vi "EVS Main.vi"() -> ()   [LabVIEW 2009]
uses:
  TypeDefs/cRIO-EVS Comm/EVS to cRIO UDP packet.ctl
  UDP Lib/UDP Network Location.ctl
  <vilib>/vision/driver/NI_Vision_Acquisition_Software.lvlib
  <vilib>/NI_Real-Time Target Support.lvlib
  <vilib>/Platform/TimedLoop/XDataNode/XDataNode.xnode
  <vilib>/Platform/TimedLoop/XDataNode/timing_clust.ctl
  <vilib>/Platform/TimedLoop/XDataNode/XDNodeRunTimeDep.lvlib
  <vilib>/Platform/TimedLoop/XDataNode/wakeup.ctl
  <vilib>/Platform/TimedLoop/XDataNode/nitl_modes.ctl
  <vilib>/vision/driver/IMAQdx.llb/IMAQdx Acquisition Mode.ctl
  <vilib>/Platform/TimedLoop/XDataNode/loadlvalarms.vi
  <vilib>/userDefined/High Color/IMAQdx.ctl
panel:
  out "Original":T1(plugin-control)
  out "Extracted":T1(plugin-control)
  out "Ramp?":bool
  out "Iteration Duration":i64
  out "Number of ramp regions (left)":i32
  out "Number of ramp regions (right)":i32
  out "Sick array":u16[](array[numeric])
  in  "stop":bool
  out "HB":bool
  in  "IMAQdx Session Left":T2="lcam" caption="Left Session"
  in  "IMAQdx Session Right":T2="rcam" caption="Right Session"
  # "0: Original\n1: Extracted\n2: Masked"
  # "0: Old line extraction\n1: Solid white line (ramp)\n2: LPF"
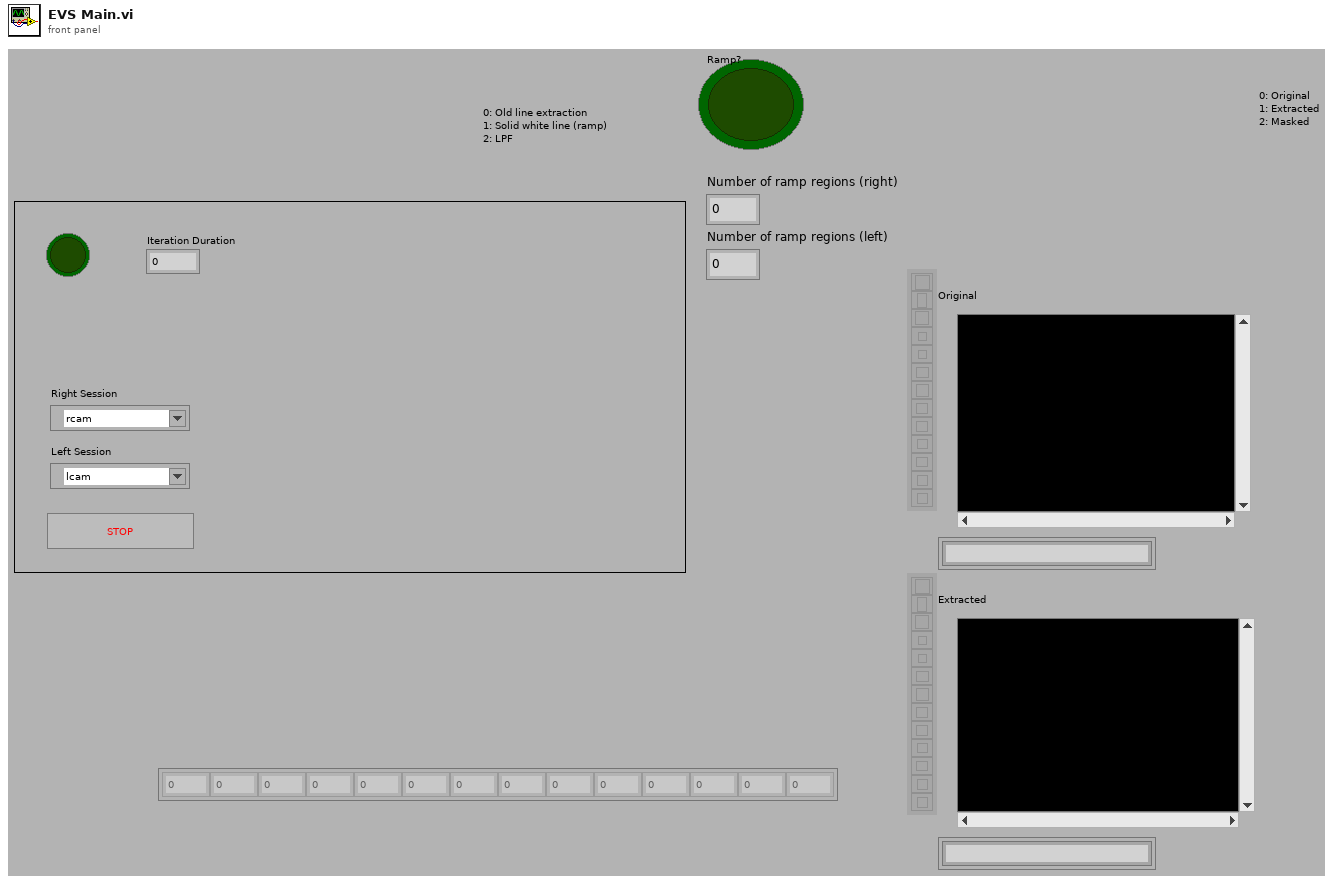
[diagram p1: front panel]
types:
  T1 = typedef "IMAQ Image.ctl" = refnum<image>
  T2 = typedef "IMAQdx.ctl" = refnum<k21>
  T3 = typedef "EVS to cRIO UDP packet.ctl" = cluster{"Camera SICK":u16[], "Camera init":bool, "Array":cluster{"X Coord":void[], "Y Coord":void[]}[]}
  T4 = typedef "NI_Vision_Acquisition_Software.lvlib/IMAQdx Acquisition Mode.ctl" = enum32{"One Shot", "Continuous"}
  T5 = typedef "XDNodeRunTimeDep.lvlib/timing_clust.ctl" = cluster{"Expected End [f-1]":u64, "Actual End [f-1]":u64, "Finished Late? [f-1]":bool, "Expected End [i-1]":u64, "Actual End [i-1]":u64, "Finished Late? [i-1]":bool, "Expected Start [i]":u64, "Actual Start [i]":u64, "Expected Start [f]":u64, "Actual Start [f]":u64, "Source Name":string, "Structure Name":string, "Period":i64, "Deadline":i64, "Offset":i64, "Start":i64, "Priority":i32, "Timeout":i32, "Mode":T6, "Wakeup Reason":T7, "Error":errorcluster, "Source Type":string, "Secondary Source Type":string, "Global End Time":u64, "Global Start Time":u64, "Frame Duration":u64, "Iteration Duration":u64, "Assigned CPU":i32, "I/O Scan Engine Mode":u32}
  T6 = typedef "XDNodeRunTimeDep.lvlib/nitl_modes.ctl" = enum32{"No Change", "Process missed periods, maintain original phase", "Discard missed periods, maintain original phase", "Process missed periods, ignore original phase", "Discard missed periods, ignore original phase"}
  T7 = typedef "XDNodeRunTimeDep.lvlib/wakeup.ctl" = enum32{"Normal", "Aborted", "Asynchronous wakeup", "Timing source error", "Timed loop error", "Timeout"}
  T8 = typedef "UDP Network Location.ctl" = cluster{"IP Address":string, "Port":u16}
  T9 = typedef "UDP Base.ctl" = cluster{"UDP Session":refnum<k16>, "UDP Socket Params":T10}
  T10 = typedef "UDP Socket Params.ctl" = cluster{"Local Port":u16, "Read Timeout":i32, "Write Timeout":i32}
  T11 = typedef "Image Type" = u32
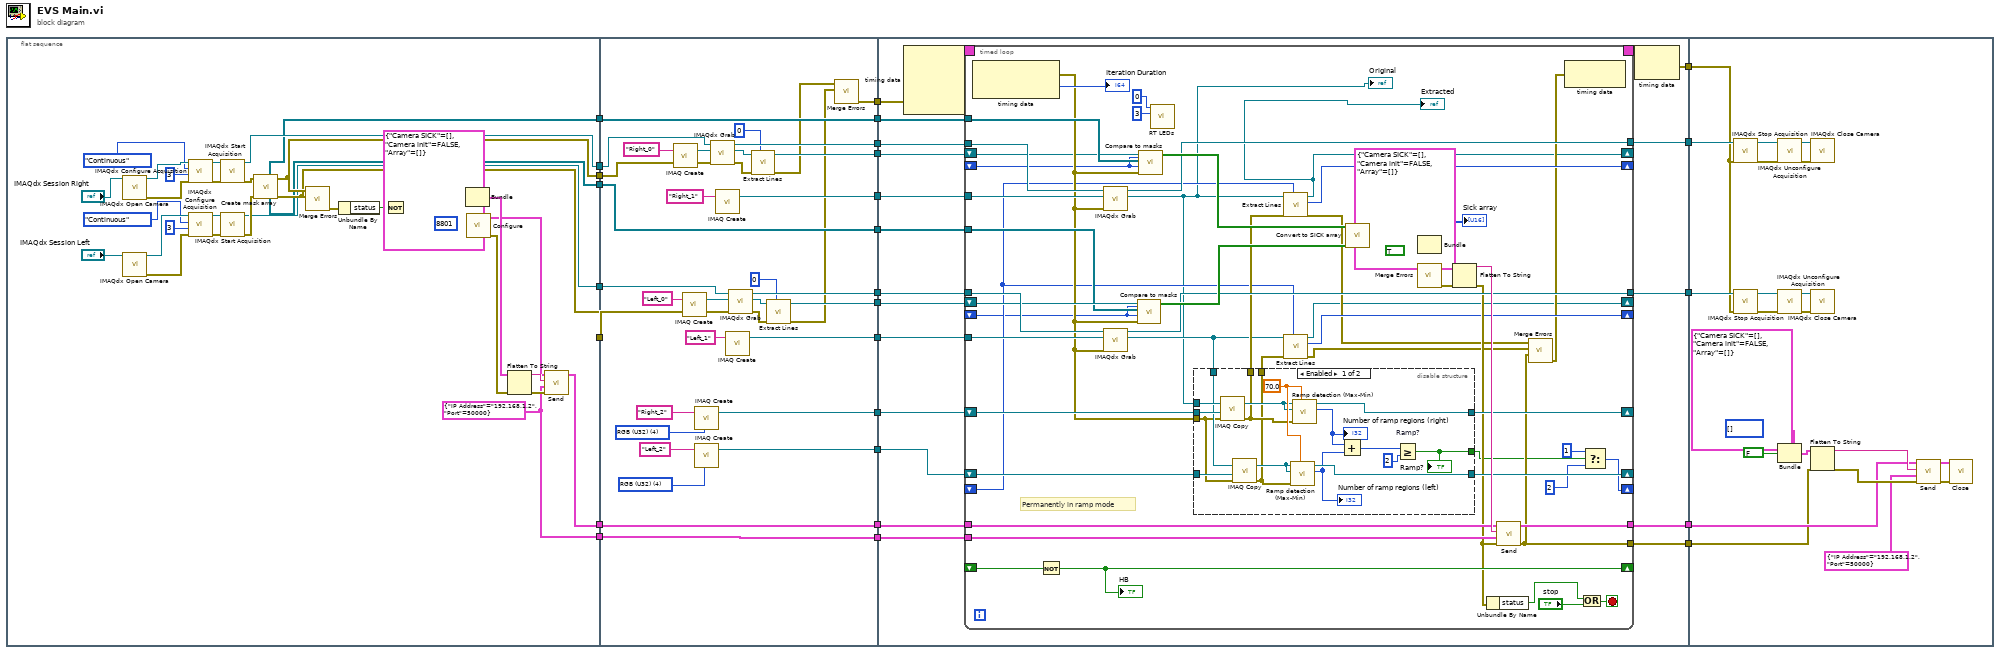
[diagram p0: block diagram]
diagram:
  n1 = flat-sequence {
    tunnel: [w40] -> w26
    tunnel: [w39] -> w25
    tunnel: [w38] -> w24
    tunnel: [w37] -> w23
    tunnel: [w36] -> w16
    tunnel: [w35] -> w14
    tunnel: [w34] -> w13
    tunnel: [w30] -> w5
    tunnel: w26 -> [w89]
    tunnel: w25 -> [w88]
    tunnel: w24 -> [w85]
    tunnel: w23 -> [w84]
    tunnel: [w83] -> w22
    tunnel: [w80] -> w21
    tunnel: [w79] -> w20
    tunnel: [w78] -> w19
    tunnel: [w77] -> w18
    tunnel: [w76] -> w17
    tunnel: w16 -> [w75]
    tunnel: [w75] -> w15
    tunnel: w14 -> [w74]
    tunnel: w13 -> [w73]
    tunnel: [w74] -> w12
    tunnel: [w73] -> w11
    tunnel: [w72] -> w6
    tunnel: w5 -> [w72]
    tunnel: [w69] -> w4
    tunnel: [w68] -> w3
    tunnel: [w65] -> w2
    tunnel: w22 -> [w106]
    tunnel: w21 -> [w105]
    tunnel: w20 -> [w117]
    tunnel: w19 -> [w116]
    tunnel: w18 -> [w115]
    tunnel: w17 -> [w114]
    tunnel: w15 -> [w113]
    tunnel: w12 -> [w112]
    tunnel: w11 -> [w111]
    tunnel: [w110] -> w10
    tunnel: [w109] -> w9
    tunnel: [w108] -> w8
    tunnel: [w107] -> w7
    tunnel: w6 -> [w104]
    tunnel: w4 -> [w101]
    tunnel: w3 -> [w100]
    tunnel: w2 -> [w99]
    tunnel: [w98] -> w1
    tunnel: w10 -> [w213]
    tunnel: w9 -> [w212]
    tunnel: w8 -> [w208]
    tunnel: w7 -> [w207]
    tunnel: w1 -> [w200]
    frame #0 {
      w30 = T8 {"IP Address"="192.168.1.2", "Port"=50000} ("cRIO Network Location")
      n2 = call <vilib>:"IMAQdx Open Camera.vi"("Session In"="IMAQdx Session Right") -> ("error out"=w59:errorcluster, "Session Out"=w58:T2)  [unwired: 2 in, 7 out]
      n3 = call <vilib>:"IMAQdx Open Camera.vi"("Session In"="IMAQdx Session Left") -> ("error out"=w53:errorcluster, "Session Out"=w54:T2)  [unwired: 2 in, 7 out]
      n4 = call <vilib>:"IMAQdx Configure Acquisition.vi"("error in"=w59, "Number of Buffers"=u32 3, "Continuous?"=IMAQdx_Acquisition_Mode."Continuous", "Session In"=w58) -> ("error out"=w60:errorcluster, "Session Out"=w57:T2)  [unwired: 1 in, 5 out]
      n5 = call <vilib>:"IMAQdx Configure Acquisition.vi"("error in"=w53, "Number of Buffers"=u32 3, "Continuous?"=IMAQdx_Acquisition_Mode."Continuous", "Session In"=w54) -> ("error out"=w52:errorcluster, "Session Out"=w55:T2)  [unwired: 1 in, 5 out]
      n6 = call <vilib>:"IMAQdx Start Acquisition.vi"("error in"=w60, "Session In"=w57) -> ("error out"=w46:errorcluster, "Session Out"=w37:T2)  [unwired: 8 out]
      n7 = call <vilib>:"IMAQdx Start Acquisition.vi"("error in"=w52, "Session In"=w55) -> ("error out"=w45:errorcluster, "Session Out"=w38:T2)  [unwired: 8 out]
      n8 = call "Create mask array.vi"("Left error in"=w45, "Right Error in"=w46) -> ("Left error out"=w39:errorcluster, "Right error out"=w40:errorcluster, "Left Cam Masks"=w34:T1[], "Right Cam Masks"=w35:T1[])  [unwired: 6 in]
      n9 = call <vilib>:"Merge Errors.vi"("error in 2 (no error)"=w39, "error in 1 (no error)"=w40) -> ("error out"=w31:errorcluster)  [unwired: 5 in]
      n10 = Unbundle By Name(w31) -> ("status"=w44:bool)
      n11 = Not(x=w44) -> (.not. x?=w32:bool)
      n12 = Bundle(cluster=T3 {"Camera SICK"=[], "Camera init"=FALSE, "Array"=[]} ("EVS to cRIO UDP packet"), "Camera init"=w32) -> (w43:T3)  [unwired: 2 in]
      n13 = call "Configure.vi"("Local Port"=u16 8801) -> ("error out"=w27:errorcluster, "UDP Base out"=w28:T9)  [unwired: 9 in]
      n14 = Flatten To String(anything=w43, error in (no error)=w27) -> (data string=w42:string, error out=w41:errorcluster)  [unwired: 2 in, 1 out]
      n15 = call "Send.vi"("error in (no error)"=w41, "Destination Location"=w30, "Send Data"=w42, "UDP Base in"=w28) -> ("UDP Base out"=w36:T9)  [unwired: 5 in, 2 out]
    }
    frame #1 {
      w63 = T11 4 items=["Grayscale (U8)", "Grayscale (I16)", "Grayscale (SGL)", "Complex (CSG)", "RGB (U32)", "HSL (U32)", "RGB (U64)", "Grayscale (U16)"] ("Image Type")
      w64 = T11 4 items=["Grayscale (U8)", "Grayscale (I16)", "Grayscale (SGL)", "Complex (CSG)", "RGB (U32)", "HSL (U32)", "RGB (U64)", "Grayscale (U16)"] ("Image Type")
      n16 = call "IMAQ Create"("Image Name"="Right_0", "error in (no error)"=w89) -> ("New Image"=w91:T1, "error out"=w90:errorcluster)  [unwired: 3 in]
      n17 = call "IMAQ Create"("Image Name"="Left_0", "error in (no error)"=w88) -> ("New Image"=w93:T1, "error out"=w92:errorcluster)  [unwired: 3 in]
      n18 = call "IMAQ Create"("Image Name"="Right_2", "Image Type"=w64) -> ("New Image"=w69:T1)  [unwired: 3 in, 1 out]
      n19 = call "IMAQ Create"("Image Name"="Left_2", "Image Type"=w63) -> ("New Image"=w68:T1)  [unwired: 3 in, 1 out]
      n20 = call <vilib>:"IMAQdx Grab.vi"("error in"=w90, "Image In"=w91, "Session In"=w84) -> ("error out"=w97:errorcluster, "Image Out"=w94:T1, "Session Out"=w79:T2)  [unwired: 5 in, 1 out]
      n21 = call "IMAQ Create"("Image Name"="Right_1") -> ("New Image"=w83:T1)  [unwired: 4 in, 1 out]
      n22 = call "IMAQ Create"("Image Name"="Left_1") -> ("New Image"=w80:T1)  [unwired: 4 in, 1 out]
      n23 = call <vilib>:"IMAQdx Grab.vi"("error in"=w92, "Image In"=w93, "Session In"=w85) -> ("error out"=w96:errorcluster, "Image Out"=w95:T1, "Session Out"=w78:T2)  [unwired: 5 in, 1 out]
      n24 = call "Extract Lines.vi"("Extraction mode"=0, "error in (no error)"=w97, "Image Src"=w94) -> ("error out"=w67:errorcluster, "Image Out"=w77:T1)  [unwired: 6 in, 1 out]
      n25 = call "Extract Lines.vi"("Extraction mode"=0, "error in (no error)"=w96, "Image Src"=w95) -> ("error out"=w66:errorcluster, "Image Out"=w76:T1)  [unwired: 6 in, 1 out]
      n26 = call <vilib>:"Merge Errors.vi"("error in 2 (no error)"=w66, "error in 1 (no error)"=w67) -> ("error out"=w65:errorcluster)  [unwired: 5 in]
    }
    frame #2 {
      n27 = node-c288(w99) -> (w103:T5)  [unwired: 3 in]
      n28 = timed-loop {
        tunnel: w117 -> [w171]
        tunnel: w116 -> [w170]
        shift-right: [w121] -> _
        shift-left: w115 -> [w122]
        shift-right: [w124] -> _
        shift-left: w114 -> [w169]
        shift-right: [w140] -> _
        shift-left: _ -> [w118]
        shift-right: [w141] -> _
        shift-left: _ -> [w119]
        tunnel: w113 -> [w165]
        tunnel: [w164] -> w108
        tunnel: [w134] -> w107
        tunnel: w112 -> [w163]
        tunnel: w111 -> [w162]
        tunnel: [w161] -> w109
        tunnel: [w160] -> w110
        tunnel: w106 -> [w159]
        tunnel: w105 -> [w158]
        tunnel: w104 -> [w153]
        shift-right: [w152] -> _
        shift-left: _ -> [w151]
        timing: w103 -> [_]
        timing-out: [_] -> w102
        shift-right: [w147] -> _
        shift-left: w101 -> [w139]
        shift-right: [w146] -> _
        shift-left: w100 -> [w138]
        shift-right: [w125] -> _
        shift-left: _ -> [w129]
        stop <- w145 stop-if-true
        # "Permanently in ramp mode"
        n29 = node-c288() -> (w137:errorcluster, →"Iteration Duration":i64)  [unwired: 1 in]
        n30 = Not(x=w151) -> (.not. x?=w152:bool)
        "HB" <- w152
        n31 = call <vilib>:"IMAQdx Grab.vi"("error in"=w137, "Image In"=w159, "Session In"=w171) -> ("Image Out"=w120:T1, "Session Out"=w161:T2)  [unwired: 5 in, 2 out]
        "Original" <- w120
        n32 = call <vilib>:"IMAQdx Grab.vi"("error in"=w137, "Image In"=w158, "Session In"=w170) -> ("Image Out"=w123:T1, "Session Out"=w160:T2)  [unwired: 5 in, 2 out]
        n33 = call "Compare to masks.vi"("Number of Particles1"=w118, "error in (no error)"=w137, "Number of Particles"=w118, "Mask array"=w162, "Image Src"=w169) -> ("Marked Regions"=w167:bool[])  [unwired: 5 in, 1 out]
        n34 = call "Compare to masks.vi"("Number of Particles1"=w119, "error in (no error)"=w137, "Number of Particles"=w119, "Mask array"=w163, "Image Src"=w122) -> ("Marked Regions"=w168:bool[])  [unwired: 5 in, 1 out]
        n35 = call <vilib>:"RT LEDs.vi"("State"=3, "LED Num"=0) -> ()  [unwired: 4 in, 2 out]
        n36 = disable-structure shown="Enabled" {
          disable-tunnel: [w188 _] -> w147
          disable-tunnel: [w187 _] -> w146
          disable-tunnel: [w181 _] -> w128
          disable-tunnel: w139 -> [w180 _]
          disable-tunnel: w120 -> [w179 _]
          disable-tunnel: w123 -> [w178 _]
          disable-tunnel: w138 -> [w177 _]
          disable-tunnel: w137 -> [w176 _]
          disable-tunnel: [w173 _] -> w131
          disable-tunnel: [w172 _] -> w130
          frame #0 {
            w186 = sgl 70.0 ("Tolerance")
            n37 = call "IMAQ Copy"("error in (no error)"=w176, "Image Dst"=w180, "Image Src"=w179) -> ("error out"=w173:errorcluster, "Image Dst Out"=w175:T1)  [unwired: 3 in]
            n38 = call "IMAQ Copy"("error in (no error)"=w176, "Image Dst"=w177, "Image Src"=w178) -> ("error out"=w172:errorcluster, "Image Dst Out"=w174:T1)  [unwired: 3 in]
            n39 = call "Ramp detection (Max-Min).vi"("Tolerance"=w186, "error in (no error)"=w172, "Image Dst"=w174, "Image Src"=w174) -> ("Number of ramp regions"=w184:i32, "Image Out"=w187:T1)  [unwired: 5 in, 1 out]
            "Number of ramp regions (left)" <- w184
            n40 = call "Ramp detection (Max-Min).vi"("Tolerance"=w186, "error in (no error)"=w173, "Image Dst"=w175, "Image Src"=w175) -> ("Number of ramp regions"=w185:i32, "Image Out"=w188:T1)  [unwired: 5 in, 1 out]
            "Number of ramp regions (right)" <- w185
            n41 = Add(x=w185, y=w184) -> (x+y=w183:i32)
            n42 = Greater Or Equal? "Ramp?"(x=w183, y=2) -> (x >= y?=w181:bool)
            "Ramp?" <- w181
          }
          frame #1 {
          }
        }
        n43 = call "Extract Lines.vi"("Extraction mode"=w129, "error in (no error)"=w131, "Image Src"=w120) -> ("error out"=w133:errorcluster, "Number of Particles1"=w141:i32, "Image Out"=w121:T1)  [unwired: 6 in]
        "Extracted" <- w121
        n44 = call "Extract Lines.vi"("Extraction mode"=w129, "error in (no error)"=w130, "Image Src"=w123) -> ("error out"=w132:errorcluster, "Number of Particles1"=w140:i32, "Image Out"=w124:T1)  [unwired: 6 in]
        n45 = call "Convert to SICK array.vi"("Left Regions"=w167, "Right Regions"=w168) -> ("Sick array"=w136:u16[])  [unwired: 9 in]
        "Sick array" <- w136
        n46 = call <vilib>:"Merge Errors.vi"() -> ("error out"=w143:errorcluster)  [unwired: 7 in]
        n47 = Bundle(cluster=T3 {"Camera SICK"=[], "Camera init"=FALSE, "Array"=[]} ("EVS to cRIO UDP packet"), "Camera SICK"=w136, "Camera init"=TRUE) -> (w154:T3)  [unwired: 1 in]
        n48 = Flatten To String(anything=w154, error in (no error)=w143) -> (data string=w166:string, error out=w142:errorcluster)  [unwired: 2 in, 1 out]
        n49 = Unbundle By Name(w142) -> ("status"=w157:bool)
        n50 = call "Send.vi"("error in (no error)"=w142, "Destination Location"=w153, "Send Data"=w166, "UDP Base in"=w165) -> ("error out"=w134:errorcluster, "UDP Base out"=w164:T9)  [unwired: 5 in, 1 out]
        n51 = call <vilib>:"Merge Errors.vi"("error in 3 (no error)"=w134, "error in 2 (no error)"=w132, "error in 1 (no error)"=w133) -> ("error out"=w135:errorcluster)  [unwired: 4 in]
        n52 = node-c288(w135) -> ()  [unwired: 1 out]
        n53 = Or(x=w157, y="stop") -> (x .or. y?=w145:bool)
        n54 = Select(t=1, s=w128, f=2 ("Extraction mode")) -> (s? t:f=w125:i32)
      }
      n55 = node-c288(w102) -> (w98:errorcluster)
    }
    frame #3 {
      n56 = call <vilib>:"IMAQdx Stop Acquisition.vi"("error in"=w200, "Session In"=w212) -> ("error out"=w219:errorcluster, "Session Out"=w218:T2)  [unwired: 8 out]
      n57 = call <vilib>:"IMAQdx Stop Acquisition.vi"("error in"=w200, "Session In"=w213) -> ("error out"=w215:errorcluster, "Session Out"=w214:T2)  [unwired: 8 out]
      n58 = call <vilib>:"IMAQdx Unconfigure Acquisition.vi"("error in"=w219, "Session In"=w218) -> ("error out"=w220:errorcluster, "Session Out"=w221:T2)  [unwired: 8 out]
      n59 = call <vilib>:"IMAQdx Unconfigure Acquisition.vi"("error in"=w215, "Session In"=w214) -> ("error out"=w216:errorcluster, "Session Out"=w217:T2)  [unwired: 8 out]
      n60 = Bundle(cluster=T3 {"Camera SICK"=[], "Camera init"=FALSE, "Array"=[]} ("EVS to cRIO UDP packet"), "Camera SICK"=u16[] [], "Camera init"=FALSE) -> (w202:T3)  [unwired: 1 in]
      n61 = call <vilib>:"IMAQdx Close Camera.vi"("error in"=w220, "Session In"=w221) -> ()  [unwired: 10 out]
      n62 = call <vilib>:"IMAQdx Close Camera.vi"("error in"=w216, "Session In"=w217) -> ()  [unwired: 10 out]
      n63 = Flatten To String(anything=w202, error in (no error)=w207) -> (data string=w211:string, error out=w210:errorcluster)  [unwired: 2 in, 1 out]
      n64 = call "Send.vi"("error in (no error)"=w210, "Destination Location"=T8 {"IP Address"="192.168.1.2", "Port"=50000}, "Send Data"=w211, "UDP Base in"=w208) -> ("error out"=w205:errorcluster, "UDP Base out"=w206:T9)  [unwired: 5 in, 1 out]
      n65 = call "Close.vi"("error in (no error)"=w205, "Cluster of class private data"=w206) -> ()  [unwired: 9 in, 1 out]
    }
  }
